vi "DCA Check Limits.vi"(6 "Colors":cluster{"Pass":u32, "Fail":u32, "Nop":u32}={"Pass"=6618880, "Fail"=16711680, "Nop"=16777226}, 8 "error in (no error)":errorcluster, 9 "Measurement Values":T6, 10 "Limits":T1[](array[typedef]), 11 "Limit Status Ref":refnum<vi>) -> (0 "error out":errorcluster, 2 "Passed?":bool, 3 "Limits and Passed?":cluster{"Limits":T1[], "Passed? Array":bool[]})   [LabVIEW 2011]
uses:
  TypeDefs/DCA Measurement Values.ctl
  TypeDefs/DCA Limit.ctl
  TypeDefs/DCA Limit Quantity.ctl
  TypeDefs/DCA Limit Comparison.ctl
  TypeDefs/DCA Limit Operation.ctl
  Test Referential Limit.ctl
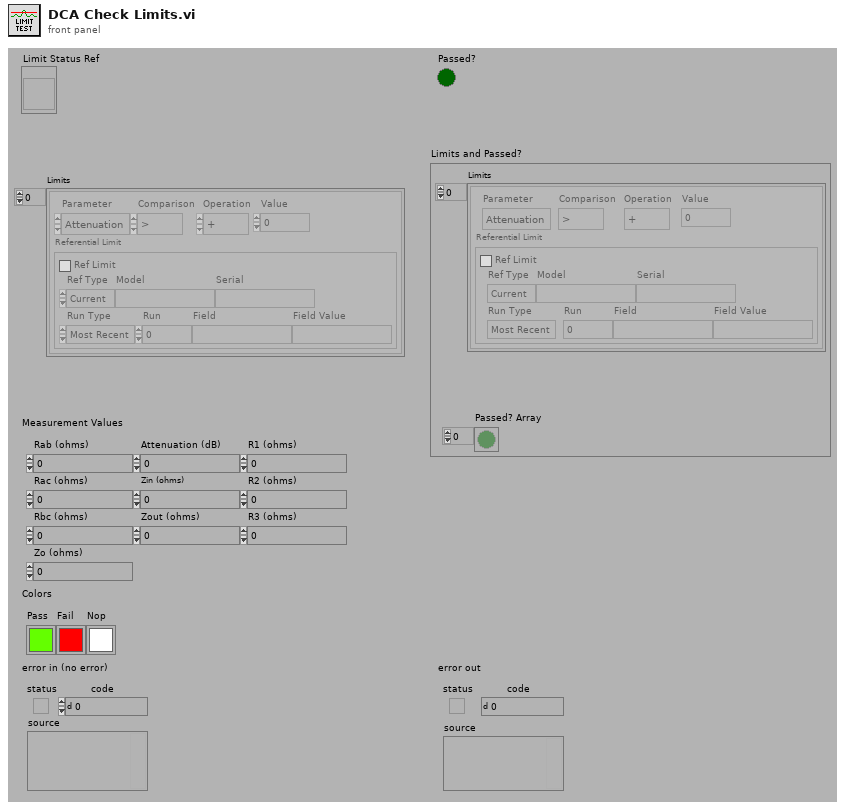
[diagram p1: front panel]
types:
  T1 = typedef "DCA Limit.ctl" = cluster{"Parameter":T2, "Comparison":T3, "Operation":T4, "Value":dbl, "Referential Limit":T5}
  T2 = typedef "DCA Limit Quantity.ctl" = enum16{"Attenuation", "Zin", "Zout", "R1", "R2", "R3", "Rab", "Rac", "Rbc"}
  T3 = typedef "DCA Limit Comparison.ctl" = enum16{">", ">=", "<", "<="}
  T4 = typedef "DCA Limit Operation.ctl" = enum16{"+", "-"}
  T5 = typedef "Test Referential Limit.ctl" = cluster{"Ref Limit":bool, "Ref Type":enum16{"Current", "Specify"}, "Model":string, "Serial":string, "Run Type":enum16{"Most Recent", "Run #", "Match Field"}, "Run":i32, "Field":string, "Field Value":string}
  T6 = typedef "DCA Measurement Values.ctl" = cluster{"Rab (ohms)":dbl, "Rac (ohms)":dbl, "Rbc (ohms)":dbl, "Zo (ohms)":dbl, "Attenuation (dB)":dbl, "Zin (ohms)":dbl, "Zout (ohms)":dbl, "R1 (ohms)":dbl, "R2 (ohms)":dbl, "R3 (ohms)":dbl}
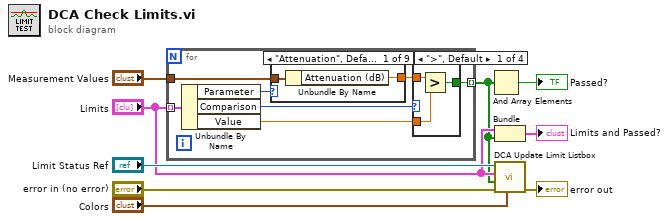
[diagram p0: block diagram]
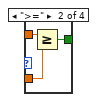
[diagram p2: hidden frame]
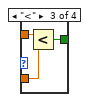
[diagram p3: hidden frame]
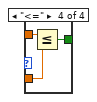
[diagram p4: hidden frame]
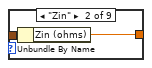
[diagram p5: hidden frame]
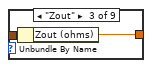
[diagram p6: hidden frame]
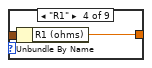
[diagram p7: hidden frame]
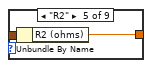
[diagram p8: hidden frame]
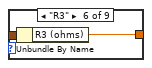
[diagram p9: hidden frame]
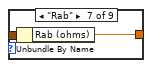
[diagram p10: hidden frame]
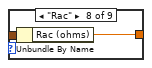
[diagram p11: hidden frame]
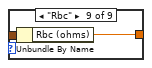
[diagram p12: hidden frame]
diagram:
  n1 = for {
    tunnel: "Limits" -> [w16] mode=indexing
    tunnel: "Measurement Values" -> [w14]
    tunnel: [w10] -> w2 mode=indexing
    n2 = Unbundle By Name(w16) -> ("Parameter"=w15:T2, "Comparison"=w13:T3, "Value"=w11:dbl)
    n3 = case shown="\"Attenuation\", Default" w15 {
      tunnel: w14 -> [w30 w32 w34 w36 w38 w40 w42 w44 w46]
      tunnel: [w29 w31 w33 w35 w37 w39 w41 w43 w45] -> w12
      frame "Attenuation", Default {
        n4 = Unbundle By Name(w30) -> ("Attenuation (dB)"=w29:dbl)
      }
      frame "Zin" {
        n5 = Unbundle By Name(w32) -> ("Zin (ohms)"=w31:dbl)
      }
      frame "Zout" {
        n6 = Unbundle By Name(w34) -> ("Zout (ohms)"=w33:dbl)
      }
      frame "R1" {
        n7 = Unbundle By Name(w36) -> ("R1 (ohms)"=w35:dbl)
      }
      frame "R2" {
        n8 = Unbundle By Name(w38) -> ("R2 (ohms)"=w37:dbl)
      }
      frame "R3" {
        n9 = Unbundle By Name(w40) -> ("R3 (ohms)"=w39:dbl)
      }
      frame "Rab" {
        n10 = Unbundle By Name(w42) -> ("Rab (ohms)"=w41:dbl)
      }
      frame "Rac" {
        n11 = Unbundle By Name(w44) -> ("Rac (ohms)"=w43:dbl)
      }
      frame "Rbc" {
        n12 = Unbundle By Name(w46) -> ("Rbc (ohms)"=w45:dbl)
      }
    }
    n13 = case shown="\">\", Default" w13 {
      tunnel: w12 -> [w19 w22 w25 w28]
      tunnel: w11 -> [w18 w21 w24 w27]
      tunnel: [w17 w20 w23 w26] -> w10
      frame ">", Default {
        n14 = Greater?(x=w19, y=w18) -> (0:w17:bool)
      }
      frame ">=" {
        n15 = Greater Or Equal?(x=w22, y=w21) -> (x >= y?=w20:bool)
      }
      frame "<" {
        n16 = Less?(x=w25, y=w24) -> (x < y?=w23:bool)
      }
      frame "<=" {
        n17 = Less Or Equal?(x=w28, y=w27) -> (x <= y?=w26:bool)
      }
    }
  }
  n18 = And Array Elements(Boolean array=w2) -> (logical AND=→"Passed?":bool)
  n19 = Bundle("Limits"="Limits", w2) -> (→"Limits and Passed?":cluster{"Limits":T1[], bool[]})  [unwired: 1 out]
  n20 = call "DCA Update Limit Listbox.vi"("Colors"="Colors", "error in (no error)"="error in (no error)", "Pass/Fail"=w2, "Limits"="Limits", "Limit Status Ref"="Limit Status Ref") -> ("error out"=→"error out":errorcluster)  [unwired: 1 in, 5 out]
